vi "Read UI Constants.vi"(8 "error in":errorcluster, 11 "CFG File Refnum in":T1) -> (0 "error out":errorcluster, 2 "MHL Configuration":T2, 3 "CFG File Refnum out":T1)   [LabVIEW 2021]
uses:
  <vilib>/Utility/config.llb/Config Data RefNum.ctl
  controls/MHL Configuration.ctl
  Boiler System Globals.vi
  <vilib>/Utility/config.llb/Read Key (Double).vi
  <vilib>/Utility/config.llb/NI_LVConfig.lvlib
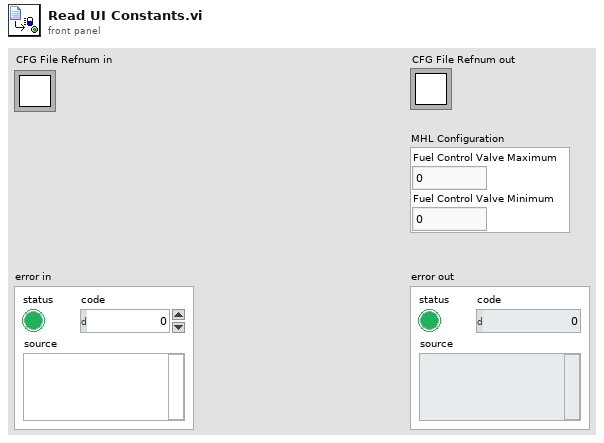
[diagram p1: front panel]
types:
  T1 = typedef "NI_LVConfig.lvlib/Config Data RefNum.ctl" = refnum<k1>
  T2 = typedef "MHL Configuration.ctl" = cluster{"Fuel Control Valve Maximum":dbl, "Fuel Control Valve Minimum":dbl}
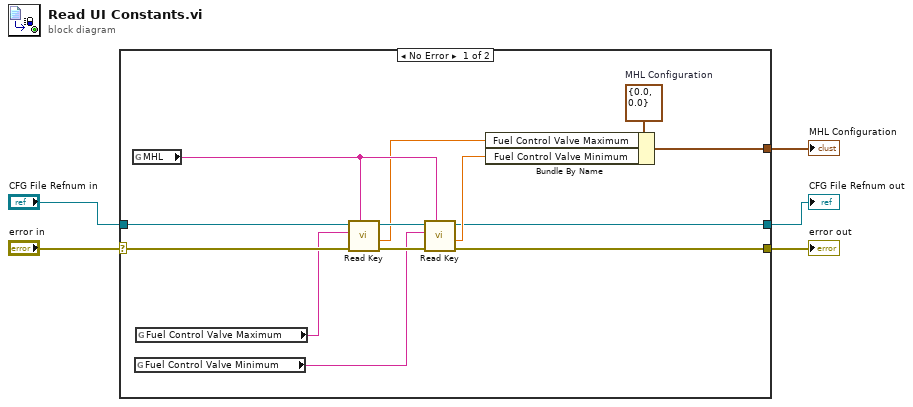
[diagram p0: block diagram]
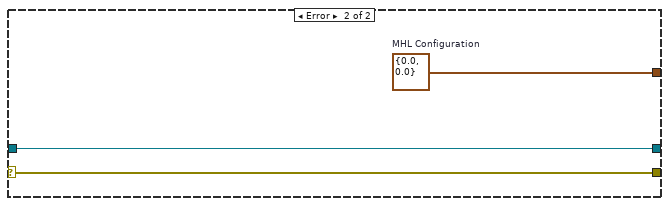
[diagram p2: hidden frame]
diagram:
  n1 = case shown="No Error" "error in" {
    selector: "error in" -> [w18 w19]
    tunnel: [w16 w19] -> w4
    tunnel: "CFG File Refnum in" -> [w14 w20]
    tunnel: [w7 w21] -> w2
    tunnel: [w6 w20] -> w1
    frame No Error {
      w9 = T2 {"Fuel Control Valve Maximum"=0.0, "Fuel Control Valve Minimum"=0.0}  # MHL Configuration
      n2 = global read "Boiler System Globals.vi" "MHL"() -> (w15:string)
      n3 = global read "Boiler System Globals.vi" "Fuel Control Valve Minimum"() -> (w12:string)
      n4 = global read "Boiler System Globals.vi" "Fuel Control Valve Maximum"() -> (w13:string)
      n5 = call-poly <vilib>:"Read Key.vi"("section"=w15, "error in (no error)"=w18, "key"=w13, "refnum"=w14) -> ("error out"=w17:errorcluster, "value"=w10:dbl, "refnum out"=w11:T1)  [unwired: 4 in, 1 out]
      n6 = call-poly <vilib>:"Read Key.vi"("section"=w15, "error in (no error)"=w17, "key"=w12, "refnum"=w11) -> ("error out"=w16:errorcluster, "value"=w8:dbl, "refnum out"=w6:T1)  [unwired: 4 in, 1 out]
      n7 = Bundle By Name(cluster=w9, "Fuel Control Valve Maximum"=w10, "Fuel Control Valve Minimum"=w8) -> (w7:T2)
    }
    frame Error {
      w21 = T2 {"Fuel Control Valve Maximum"=0.0, "Fuel Control Valve Minimum"=0.0}  # MHL Configuration
    }
  }
  "error out" <- w4
  "MHL Configuration" <- w2
  "CFG File Refnum out" <- w1
